vi "tcpMessageClient.vi"(11 "client configuration":T2={"client ID"="tcpClient", "remote host"="localhost", "local port"=50000, "remote port"=50001}) -> (0 "error out":errorcluster)   [LabVIEW 2014]
doc: "A couple tcpMessageServer and tcpMessageClient ensures communication between two instances. Each one can both transmit or receive CR/LF terminated message strings; however one of the member has to be a Server and the other a Client. Both sit and wait for the other party to connect.\n\nThe difference is: \n* the Server accpts connections on the specified port from any incoming host (the inputs \"remote host\" and \"remote port\" are ignored) \n* the Client must know to which host is directed\n\nCommunication with them, while running, is done via four named queues. One acts as a transmission buffer, another as a receive buffer; one is a single element queue, which cause the shutdown of the actor when a True is enqueued to it; the last one is a read only one-element queue which reports the actor status."
uses:
  typedefs/clientConfiguration.ctl
  typedefs/clientStatus.ctl
panel:
  in  "manual shutdown":bool
  out "status":T1
  out "received string":string
  out "string to send":string
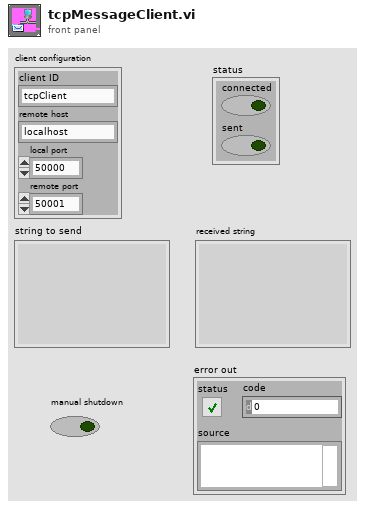
[diagram p1: front panel]
types:
  T1 = typedef "clientStatus.ctl" = cluster{"connected":bool, "sent":bool}
  T2 = typedef "clientConfiguration.ctl" = cluster{"client ID":string, "remote host":string, "local port":u16, "remote port":u16}
  T3 = cluster{"status":cluster{"queue":refnum<queue>, "error out":errorcluster}, "receive":cluster{"queue":refnum<queue>, "error out":errorcluster}, "transmit":cluster{"queue":refnum<queue>, "error out":errorcluster}, "shutdown":cluster{"queue":refnum<queue>, "error out":errorcluster}}
  T4 = cluster{"queue":refnum<queue>, "error out":errorcluster}
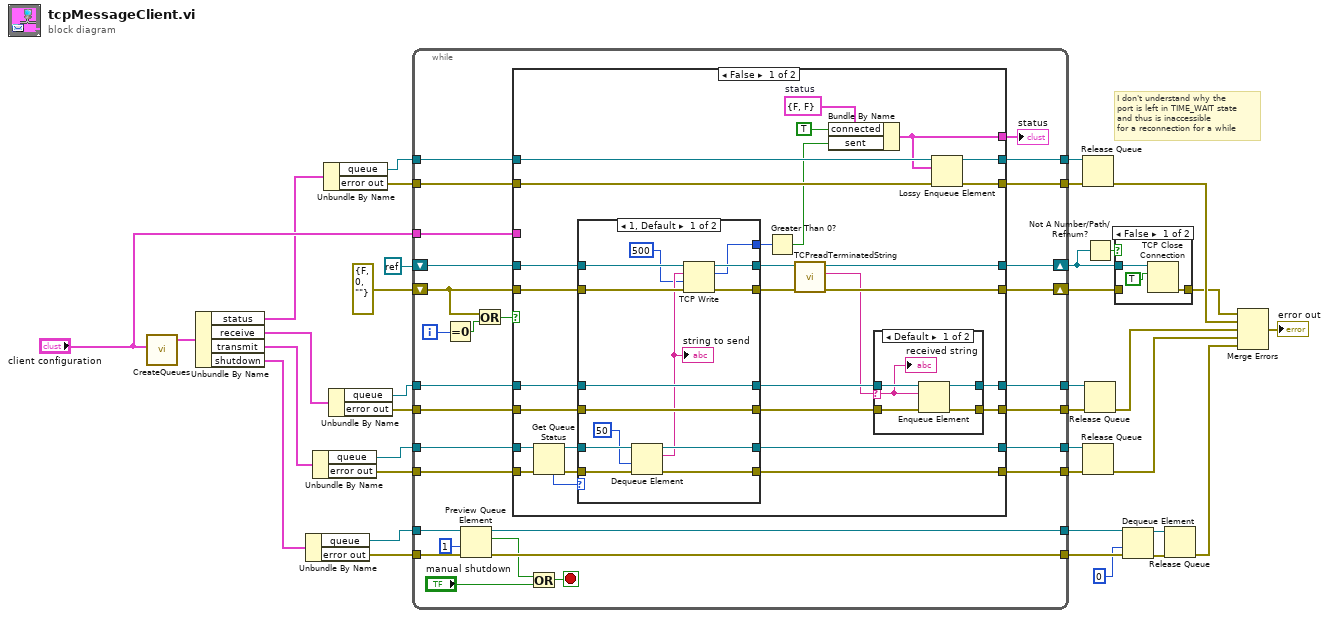
[diagram p0: block diagram]
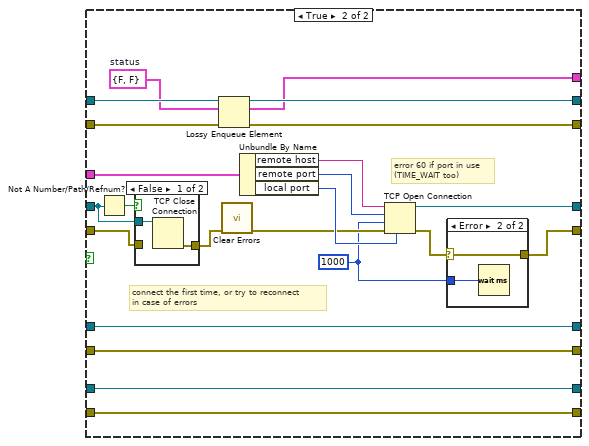
[diagram p5: hidden frame]
diagram:
  # "I don't understand why the\nport is left in TIME_WAIT state\nand thus is inaccessible\nfor a reconnection for a while"
  n1 = call "CreateQueues.vi"("client configuration"="client configuration") -> ("output cluster"=w11:T3)  [unwired: 10 in]
  n2 = Unbundle By Name(w11) -> ("status"=w14:T4, "receive"=w17:T4, "transmit"=w18:T4, "shutdown"=w23:T4)
  n3 = Unbundle By Name(w23) -> ("queue"=w22:refnum<queue>, "error out"=w21:errorcluster)
  n4 = Unbundle By Name(w18) -> ("queue"=w19:refnum<queue>, "error out"=w20:errorcluster)
  n5 = Unbundle By Name(w14) -> ("queue"=w13:refnum<queue>, "error out"=w12:errorcluster)
  n6 = Unbundle By Name(w17) -> ("queue"=w16:refnum<queue>, "error out"=w15:errorcluster)
  n7 = while {
    shift-right: [w63] -> w8
    shift-left: errorcluster {"status"=FALSE, "code"=0, "source"=""} ("error out") -> [w62]
    shift-right: [w64] -> w9
    shift-left: refnum<k0> refnum -> [w65]
    tunnel: "client configuration" -> [w58]
    tunnel: w21 -> [w43]
    tunnel: w22 -> [w44]
    tunnel: w13 -> [w57]
    tunnel: w12 -> [w56]
    tunnel: w16 -> [w55]
    tunnel: w15 -> [w54]
    tunnel: w19 -> [w53]
    tunnel: w20 -> [w52]
    tunnel: [w42] -> w5
    tunnel: [w41] -> w3
    tunnel: [w51] -> w35
    tunnel: [w50] -> w34
    tunnel: [w48] -> w33
    tunnel: [w47] -> w32
    tunnel: [w46] -> w31
    tunnel: [w45] -> w30
    i -> [w61]
    stop <- w38 stop-if-true
    n8 = Equal To 0?(x=w61) -> (x = 0?=w60:bool)
    n9 = Preview Queue Element(queue=w44, timeout in ms (-1)=1, error in (no error)=w43) -> (queue out=w42:refnum<queue>, element=w39:bool, error out=w41:errorcluster)  [unwired: 1 out]
    n10 = Or(x=w62, y=w60) -> (x .or. y?=w59:bool)
    n11 = case shown="False" w59 {
      tunnel: w65 -> [w78 w127]
      tunnel: [w73 w139] -> w64
      tunnel: [w71 w123] -> w63
      tunnel: w62 -> [w77 w126]
      tunnel: w58 -> [_ w142]
      tunnel: w57 -> [w94 w138]
      tunnel: w56 -> [w93 w137]
      tunnel: w55 -> [w80 w133]
      tunnel: w54 -> [w79 w132]
      tunnel: w53 -> [w88 w131]
      tunnel: w52 -> [w87 w130]
      tunnel: [w92 w136] -> w51
      tunnel: [w91 w135] -> w50
      tunnel: [w83 w134] -> w49
      tunnel: [w68 w133] -> w48
      tunnel: [w67 w132] -> w47
      tunnel: [w82 w131] -> w46
      tunnel: [w81 w130] -> w45
      frame False {
        w90 = T1 {"connected"=FALSE, "sent"=FALSE}  # status
        n12 = Get Queue Status(queue=w88, error in (no error)=w87) -> (queue out=w85:refnum<queue>, error out=w84:errorcluster, # elements in queue=w86:i32)  [unwired: 1 in, 5 out]
        n13 = case shown="1, Default" w86 {
          tunnel: w85 -> [w115 w117]
          tunnel: w84 -> [w114 w116]
          tunnel: [w113 w117] -> w82
          tunnel: [w112 w116] -> w81
          tunnel: w80 -> [w111 w121]
          tunnel: w79 -> [w110 w120]
          tunnel: [w111 w121] -> w70
          tunnel: [w110 w120] -> w69
          tunnel: w78 -> [w109 w119]
          tunnel: w77 -> [w108 w118]
          tunnel: [w107 w119] -> w76
          tunnel: [w106 w118] -> w72
          tunnel: [w105 _] -> w75
          frame 1, Default {
            n14 = Dequeue Element(queue=w115, timeout in ms (-1)=50, error in (no error)=w114) -> (queue out=w113:refnum<queue>, element=w104:string, error out=w112:errorcluster)  [unwired: 1 out]
            "string to send" <- w104
            n15 = TCP Write(connection ID=w109, data in=w104, error in (no error)=w108, 9:500 ("timeout ms (25000)")) -> (connection ID out=w107:refnum<k5>, bytes written=w105:i32, error out=w106:errorcluster)
          }
          frame 0 {
          }
        }
        n16 = Greater Than 0?(x=w75) -> (x > 0?=w74:bool)
        n17 = call "TCPreadTerminatedString.vi"("error in (no error)"=w72, "TCP Network Connection in"=w76) -> ("error out"=w71:errorcluster, "string out"=w66:string, "TCP Network Connection out"=w73:refnum<k5>)  [unwired: 7 in]
        n18 = Bundle By Name(cluster=w90, "connected"=TRUE, "sent"=w74) -> (w83:T1)
        n19 = case shown="Default" w66 {
          selector: w66 -> [w95 _]
          tunnel: w70 -> [w97 w101]
          tunnel: w69 -> [w96 w100]
          tunnel: [w99 w101] -> w68
          tunnel: [w98 w100] -> w67
          frame Default {
            n20 = Enqueue Element(queue=w97, element=w95, error in (no error)=w96) -> (queue out=w99:refnum<queue>, error out=w98:errorcluster)  [unwired: 1 in, 1 out]
            "received string" <- w95
          }
          frame "" {
          }
        }
        n21 = Lossy Enqueue Element(queue=w94, element=w83, error in (no error)=w93) -> (queue out=w92:refnum<queue>, error out=w91:errorcluster)  [unwired: 2 out]
      }
      frame True {
        w134 = T1 {"connected"=FALSE, "sent"=FALSE}  # status
        w122 = 1000 ("timeout ms (60000)")
        # "error 60 if port in use\n(TIME_WAIT too)"
        # "connect the first time, or try to reconnect\nin case of errors"
        n22 = Not A Number/Path/Refnum?(number/path/refnum=w127) -> (NaN/Path/Refnum?=w128:bool)
        n23 = case shown="False" w128 {
          tunnel: w127 -> [w148 _]
          tunnel: w126 -> [_ w149]
          tunnel: [w147 w149] -> w125
          frame False {
            n24 = TCP Close Connection(connection ID=w148) -> (error out=w147:errorcluster)  [unwired: 2 in, 1 out]
          }
          frame True {
          }
        }
        n25 = Lossy Enqueue Element(queue=w138, element=w134, error in (no error)=w137) -> (queue out=w136:refnum<queue>, error out=w135:errorcluster)  [unwired: 2 out]
        n26 = call <vilib>:"Clear Errors.vi"("error in (no error)"=w125) -> ("error out"=w129:errorcluster)  [unwired: 5 in, 1 out]
        n27 = Unbundle By Name(w142) -> ("remote host"=w141:string, "remote port"=w143:u16, "local port"=w140:u16)
        n28 = TCP Open Connection(address=w141, remote port or service name=w143, timeout ms (60000)=w122, local port=w140, error in (no error)=w129) -> (connection ID=w139:refnum<k5>, error out=w124:errorcluster)
        n29 = case shown="Error" w124 {
          selector: w124 -> [w144 w146]
          tunnel: [w144 w146] -> w123
          tunnel: w122 -> [_ w145]
          frame No Error {
          }
          frame Error {
            n30 = Wait (ms)(milliseconds to wait=w145) -> ()  [unwired: 1 out]
          }
        }
      }
    }
    "status" <- w49
    n31 = Or(x=w39, y="manual shutdown") -> (x .or. y?=w38:bool)
  }
  n32 = Release Queue(queue=w35, error in (no error)=w34) -> (error out=w29:errorcluster)  [unwired: 1 in, 2 out]
  n33 = Release Queue(queue=w31, error in (no error)=w30) -> (error out=w27:errorcluster)  [unwired: 1 in, 2 out]
  n34 = Not A Number/Path/Refnum?(number/path/refnum=w9) -> (NaN/Path/Refnum?=w10:bool)
  n35 = Release Queue(queue=w33, error in (no error)=w32) -> (error out=w28:errorcluster)  [unwired: 1 in, 2 out]
  n36 = case shown="False" w10 {
    tunnel: w9 -> [w152 _]
    tunnel: w8 -> [_ w153]
    tunnel: [w151 w153] -> w7
    frame False {
      n37 = TCP Close Connection(connection ID=w152, abort (F)=TRUE) -> (error out=w151:errorcluster)  [unwired: 1 in, 1 out]
    }
    frame True {
    }
  }
  n38 = Dequeue Element(queue=w5, timeout in ms (-1)=0, error in (no error)=w3) -> (queue out=w4:refnum<queue>, error out=w2:errorcluster)  [unwired: 2 out]
  n39 = Release Queue(queue=w4, error in (no error)=w2) -> (error out=w26:errorcluster)  [unwired: 1 in, 2 out]
  n40 = Merge Errors(w7, w29, w28, w27, w26) -> (→"error out":errorcluster)
